vi "SUB_Write_GEN4_Init_data_V2_0_1 - 83.vi"(5 "Interval Time":enum16{"10ms", "33ms", "50ms"}(ring), 7 "Mode":T3, 8 "Connection Status":T1={"MAC Address"="F8:B8:54:EF:76:8D", "cnx handle"=0, "cnx flags"=5, "Address Type"=1, "Connection Interval (ms)"=8, "Timeout(ms)"=1000, "Latency"=0, "bonding handle"=255} {"Address Type" items=["Public", "Random"]}, 9 "83 tx start":bool, 10 "Cal information":T4 {"Check sum" format="%x"; "Voltage L 2.8V" format="%x"; "Voltage H 2.8V" format="%x"; "Voltage L 3.1V" format="%x"; "Acc Z_L_Cal" format="%x"; "Voltage H 3.1V" format="%x"; "Gyro Z_L_Cal" format="%x"; "Gyro Z_H_Cal" format="%x"; "Gyro Y_L_Cal" format="%x"; "Gyro Y_H_Cal" format="%x"; "Gyro X_L_Cal" format="%x"; "Gyro X_H_Cal" format="%x"; "Acc Z_H_Cal" format="%x"; "Acc Y_L_Cal" format="%x"; "Acc Y_H_Cal" format="%x"; "Acc X_L_Cal" format="%x"; "Acc X_H_Cal" format="%x"; "Packet ID" format="%x"}, 11 "Port-act 1":refnum<visa-resource-name>="COM8") -> (0 "83 checksum":u8, 1 "83 rx start":bool)   [LabVIEW 2015]
uses:
  Cluster Type/Cal information.ctl
  Type definition/write_mode.ctl
  Lib_Bled112 toolkit/type_def/connection_status_bundle.ctl
  Lib_Bled112 toolkit/type_def/address_type.ctl
  Lib_Bled112 toolkit/ble_functions/ble_write_by_handle_uint8array.vi
panel:
  in  "Delay(ms)":u32=3
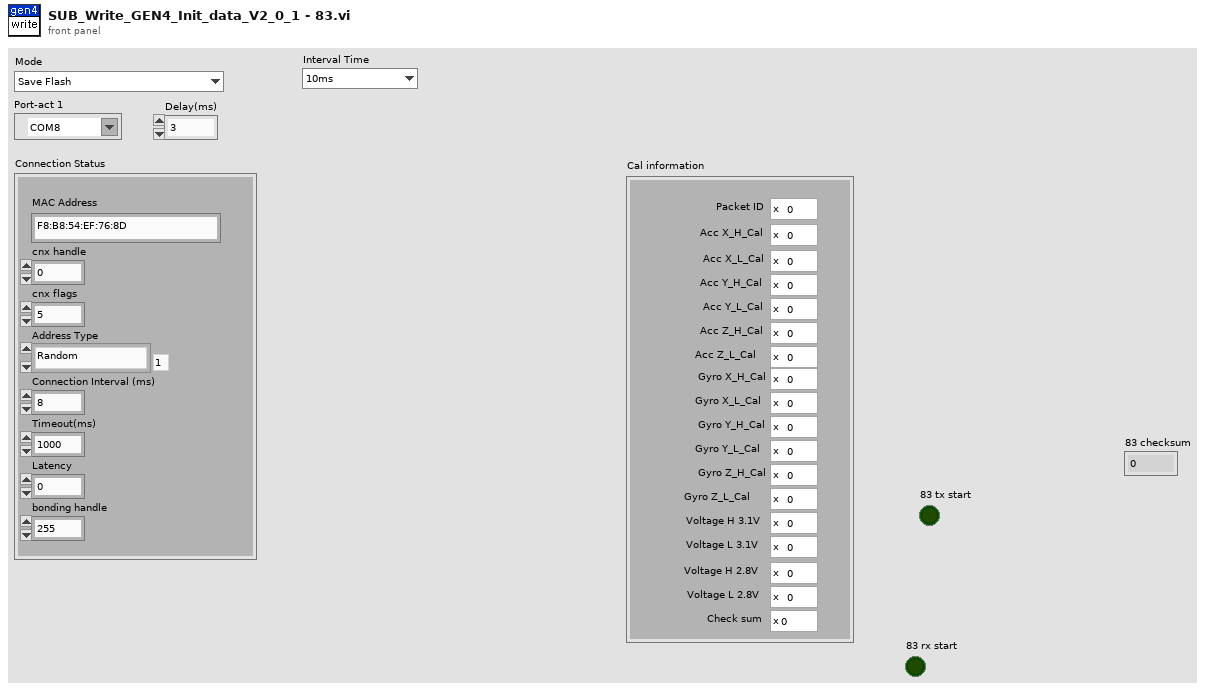
[diagram p1: front panel]
types:
  T1 = typedef "connection_status_bundle.ctl" = cluster{"MAC Address":string, "cnx handle":u8, "cnx flags":u8, "Address Type":T2, "Connection Interval (ms)":u16, "Timeout(ms)":u16, "Latency":u16, "bonding handle":u8}
  T2 = typedef "address_type.ctl" = u8
  T3 = typedef "write_mode.ctl" = enum16{"Save Flash", "Visa save", "Interval Change"}
  T4 = typedef "Cal information.ctl" = cluster{"Packet ID":u8, "Acc X_H_Cal":u8, "Acc X_L_Cal":u8, "Acc Y_H_Cal":u8, "Acc Y_L_Cal":u8, "Acc Z_H_Cal":u8, "Acc Z_L_Cal":u8, "Gyro X_H_Cal":u8, "Gyro X_L_Cal":u8, "Gyro Y_H_Cal":u8, "Gyro Y_L_Cal":u8, "Gyro Z_H_Cal":u8, "Gyro Z_L_Cal":u8, "Voltage H 3.1V":u8, "Voltage L 3.1V":u8, "Voltage H 2.8V":u8, "Voltage L 2.8V":u8, "Check sum":u8}
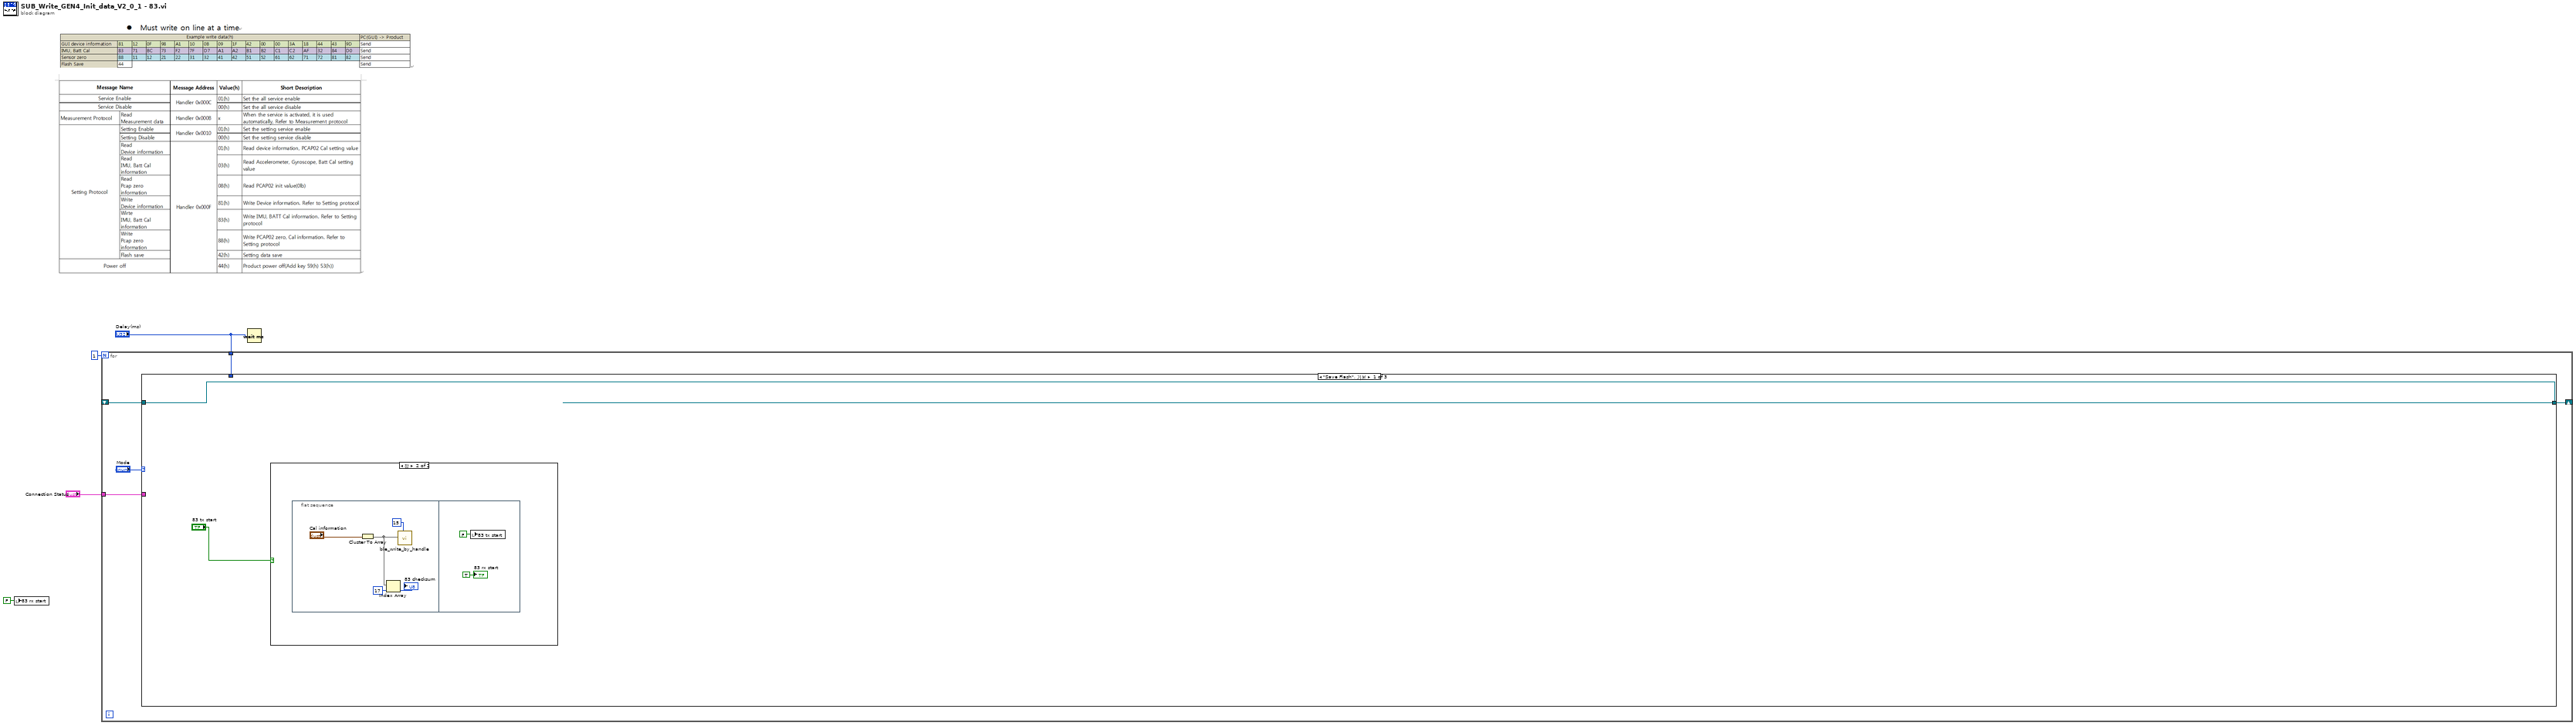
[diagram p0: block diagram]
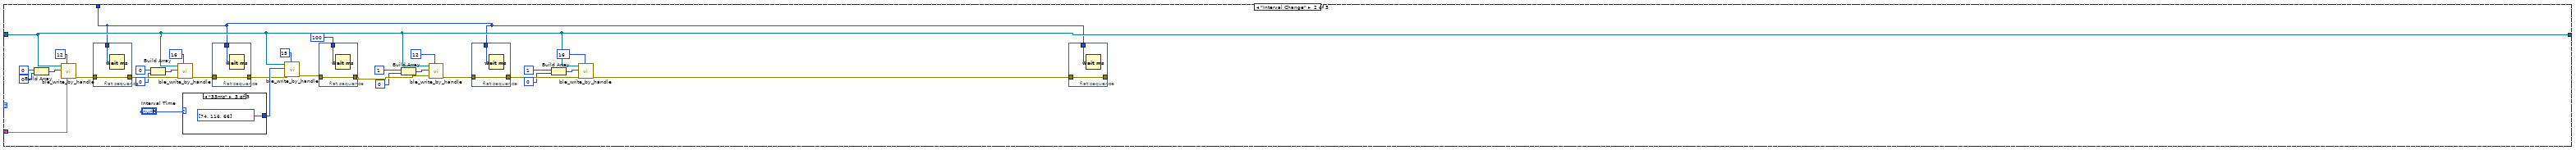
[diagram p3: hidden frame]
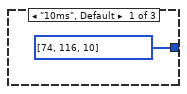
[diagram p4: hidden frame]
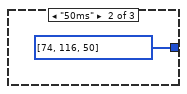
[diagram p5: hidden frame]
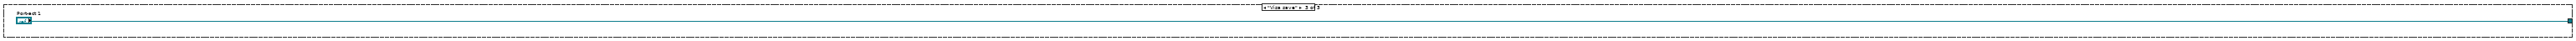
[diagram p6: hidden frame]
diagram:
  n1 = local write "83 rx start"(FALSE ("88 rx start")) -> ()
  n2 = for {
    N: 1 -> [_]
    shift-right: [w8] -> _
    shift-left: _ -> [w7]
    tunnel: "Connection Status" -> [w6]
    tunnel: "Delay(ms)" -> [w5]
    n3 = case shown="\"Save Flash\", 기본" "Mode" {
      tunnel: [w11 w36 "Port-act 1"] -> w8
      tunnel: w7 -> [w11 w36 _]
      tunnel: w6 -> [_ w49 _]
      tunnel: w5 -> [_ w24 _]
      frame "Save Flash", Default {
        n4 = case shown="참" "83 tx start" {
          frame False {
          }
          frame True {
            n5 = flat-sequence {
              frame #0 {
                n6 = Cluster To Array(cluster="Cal information") -> (array=w13:u8[])
                n7 = Index Array(array=w13, index=17 ("인덱스")) -> (element=→"83 checksum":u8)
                n8 = call-poly "ble_write_by_handle.vi"("Handle"=u16 15, "data (uint8array)"=w13) -> ()  [unwired: 8 in, 2 out]
              }
              frame #1 {
                n9 = local write "83 tx start"(FALSE ("83 tx start")) -> ()
                "83 rx start" <- TRUE ("83 rx start")
              }
            }
          }
        }
      }
      frame "Interval Change" {
        n10 = Build Array(u16 0 ("Handle"), u16 0 ("Handle")) -> (w47:u16[])
        n11 = call-poly "ble_write_by_handle.vi"("Connection Status"=w49, "Handle"=u16 12, "data (uint8array)"=w47, "COM Bluegiga in"=w36) -> ("error out"=w32:errorcluster)  [unwired: 6 in, 1 out]
        n12 = flat-sequence {
          tunnel: w24 -> [w60]
          tunnel: [w59] -> w33
          tunnel: w32 -> [w59]
          frame #0 {
            n13 = Wait (ms)(milliseconds to wait=w60) -> ()  [unwired: 1 out]
          }
        }
        n14 = Build Array(u16 0 ("Handle"), u16 0 ("Handle")) -> (w46:u16[])
        n15 = call-poly "ble_write_by_handle.vi"("Handle"=u16 16, "error in (no error)"=w33, "data (uint8array)"=w46, "COM Bluegiga in"=w36) -> ("error out"=w31:errorcluster)  [unwired: 6 in, 1 out]
        n16 = case shown="\"33ms\"" "Interval Time" {
          tunnel: [u8[] [74, 116, 10] u8[] [74, 116, 50] u8[] [74, 116, 66]] -> w34
          frame "10ms", Default {
          }
          frame "50ms" {
          }
          frame "33ms" {
          }
        }
        n17 = flat-sequence {
          tunnel: w24 -> [w58]
          tunnel: [w57] -> w30
          tunnel: w31 -> [w57]
          frame #0 {
            n18 = Wait (ms)(milliseconds to wait=w58) -> ()  [unwired: 1 out]
          }
        }
        n19 = call-poly "ble_write_by_handle.vi"("Handle"=u16 15, "error in (no error)"=w30, "data (uint8array)"=w34, "COM Bluegiga in"=w36) -> ("error out"=w29:errorcluster)  [unwired: 6 in, 1 out]
        n20 = flat-sequence {
          tunnel: u32 100 ("대기 시간(ms)") -> [w56]
          tunnel: [w55] -> w28
          tunnel: w29 -> [w55]
          frame #0 {
            n21 = Wait (ms)(milliseconds to wait=w56) -> ()  [unwired: 1 out]
          }
        }
        n22 = Build Array(u16 1 ("Handle"), u16 0 ("Handle")) -> (w40:u16[])
        n23 = call-poly "ble_write_by_handle.vi"("Handle"=u16 12, "error in (no error)"=w28, "data (uint8array)"=w40, "COM Bluegiga in"=w36) -> ("error out"=w27:errorcluster)  [unwired: 6 in, 1 out]
        n24 = flat-sequence {
          tunnel: w24 -> [w54]
          tunnel: [w53] -> w26
          tunnel: w27 -> [w53]
          frame #0 {
            n25 = Wait (ms)(milliseconds to wait=w54) -> ()  [unwired: 1 out]
          }
        }
        n26 = Build Array(u16 1 ("Handle"), u16 0 ("Handle")) -> (w41:u16[])
        n27 = call-poly "ble_write_by_handle.vi"("Handle"=u16 16, "error in (no error)"=w26, "data (uint8array)"=w41, "COM Bluegiga in"=w36) -> ("error out"=w25:errorcluster)  [unwired: 6 in, 1 out]
        n28 = flat-sequence {
          tunnel: w24 -> [w52]
          tunnel: [w51] -> _
          tunnel: w25 -> [w51]
          frame #0 {
            n29 = Wait (ms)(milliseconds to wait=w52) -> ()  [unwired: 1 out]
          }
        }
      }
      frame "Visa save" {
      }
    }
  }
  n30 = Wait (ms)(milliseconds to wait="Delay(ms)") -> ()  [unwired: 1 out]
